vi "ALLPROPS20dll.vi"(8 "error in (no error)":errorcluster, 11 "Inputs":T1) -> (0 "error out":errorcluster, 3 "Outputs":T2)   [LabVIEW 2021]
doc: "subroutine ALLPROPSdll(hOut, iUnits, iMass, iFlag, T, D, zm, Output, hUnits, iUCodeArray, ierr,\nherr, hOut_length, hUnits_length, herr_length)\n\nCalculate the single-phase properties identified in the hOut string at the temperature, density, and composition\nsent to the routine. Return the properties in mass or molar units depending on iUnits.\n\nWarning Do NOT call this routine for two-phase states, otherwise it will return metastable states if near but\ninside the phase boundary, or complete nonsense at other conditions. The value of q that is returned from the\nflash routines will indicate a two phase state by returning a value between 0 and 1. In such a situation, properties\ncan only be calculated for the saturated liquid and vapor states.\n\nFor example, when calling PHFLSH: call subroutine PHFLSH (P,h,z,T,D,Dl,Dv,x,y,q,e,s,Cv,Cp,w,ierr,herr) If q>0 and q<1,\n then values of the liquid and vapor compositions will be returned in the x and y arrays, and the properties of the \nliquid and vapor states can be calculated, for example:\n\ncall ENTRO (T,Dl,x,sliq)\ncall ENTRO (T,Dv,x,svap)\n\nINPUTS:\nhOut -- Input string of properties to calculate (of any length). Inputs can be\nseparated by spaces, commas, semicolons, or bars, but should not be mixed. For example,\na proper string would be hOut=’T,P,D,H,E,S’, whereas an improperly defined string would\nbe hOut=’T,P;D H|E,S’. Use of lower or upper case is not important. Some properties will\nreturn multiple values, for example, hOut=’F,Fc,XMOLE’ will return 12 properties for a\nfour component system, these being F(1), F(2), F(3), F(4), Fc(1), Fc(2), etc. To retrieve the\nproperty of a single component, use, for example, hOut=’XMOLE(2),XMOLE(3)’\niUnits -- See subroutine REFPROP for a complete description of the iUnits input\nvalue. A negative value for iUnits indicates that the input temperature is given in K and\ndensity in mol/dm^3, (Refprop default units), otherwise T and D will be converted first to K\nand mol/dm^3. Do not use the negative value for the iUnits parameter everywhere, only in\nthis one situation.\niMass -- Specifies if the input composition is mole or mass based.\n 0 Input compositions given in mole fractions\n 1 Input compositions given in mass fractions\niFlag -- Turn on or off writing of labels and units to hUnitsArray.\n 0 Do not write anything to the hUnitsArray array, thus increasing the calculation speed. (String handling in \n Fortran is very computationally expensive.)\n 1 Write labels and units to the hUnitsArray array.\n 2 Return only the string number described under “iUCodeArray” below and the units. (No properties will be \n calculated.)\n -1 Write labels and units for only the first item\nT -- Temperature, with units based on the value of iUnits.\nD -- Density, with units based on the value of iUnits.\nz -- Composition on a mole or mass basis (array of size ncmax=20)\n\nOUTPUTS:\nOutput -- Array of properties that were specified in the hOut string. (array\nof size 200 dimensioned as double precision) The number -9999970 will be returned when\nerrors occur or no input was requested.\nhUnits -- String with units. Will also contain error messages when necessary. The string will be empty if iFlag=0.\niUCodeArray -- Array (of size 200) with the values of iUCode(n) described\nin the REFPROP subroutine.\nierr -- Error flag\nherr -- Error string (character*255)\nhOut_length -- length of variable hOut (default: 255)\nhUnits_length -- length of variable hUnits (default: 1000)\nherr_length -- length of variable herr (default: 255)\n\nThe dimension statements for these variables are (in Fortran):\nparameter (ncmax=20) ! Maximum number of components in the mixture\nparameter (iPropMax=200) ! Number of output properties available in ALLPROPS.\ncharacter*10000 hOut ! hOut can actually be of any length.\ncharacter herr*255,hUnitsArray(iPropMax)*50\ninteger ierr,iUnits,iMass,iFlag,iUCodeArray(iPropMax) ! Note: as integer*4\ndouble precision Tx,Dx,zm(ncmax),Output(iPropMax)"
uses:
  REFPROP.dll
panel:
  # "REFPROP-ALLPROPS20dll"
  # "void  ALLPROPS20dll(CStr hOut, int32_t *iUnits, int32_t *iMass, int32_t *iFlag, double *T, double *D, double *z, double *Output, CStr hUnits, int32_t *iUCodeArray, int32_t *ierr, CStr herr, int32_t *hOut_Length, int32_t *hUnitsArray_length, int32_t *herr_length);"
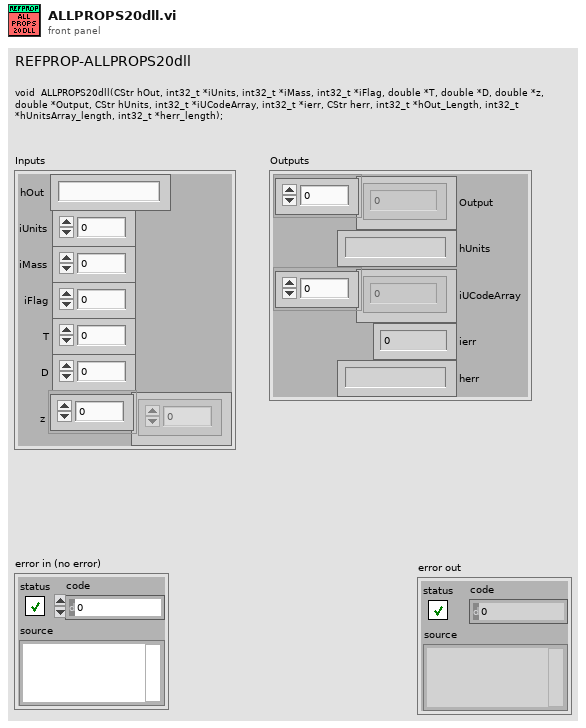
[diagram p1: front panel]
types:
  T1 = cluster{"hOut":string, "iUnits":i32, "iMass":i32, "iFlag":i32, "T":dbl, "D":dbl, "z":dbl[]}
  T2 = cluster{"Output":dbl[], "hUnits":string, "iUCodeArray":i32[], "ierr":i32, "herr":string}
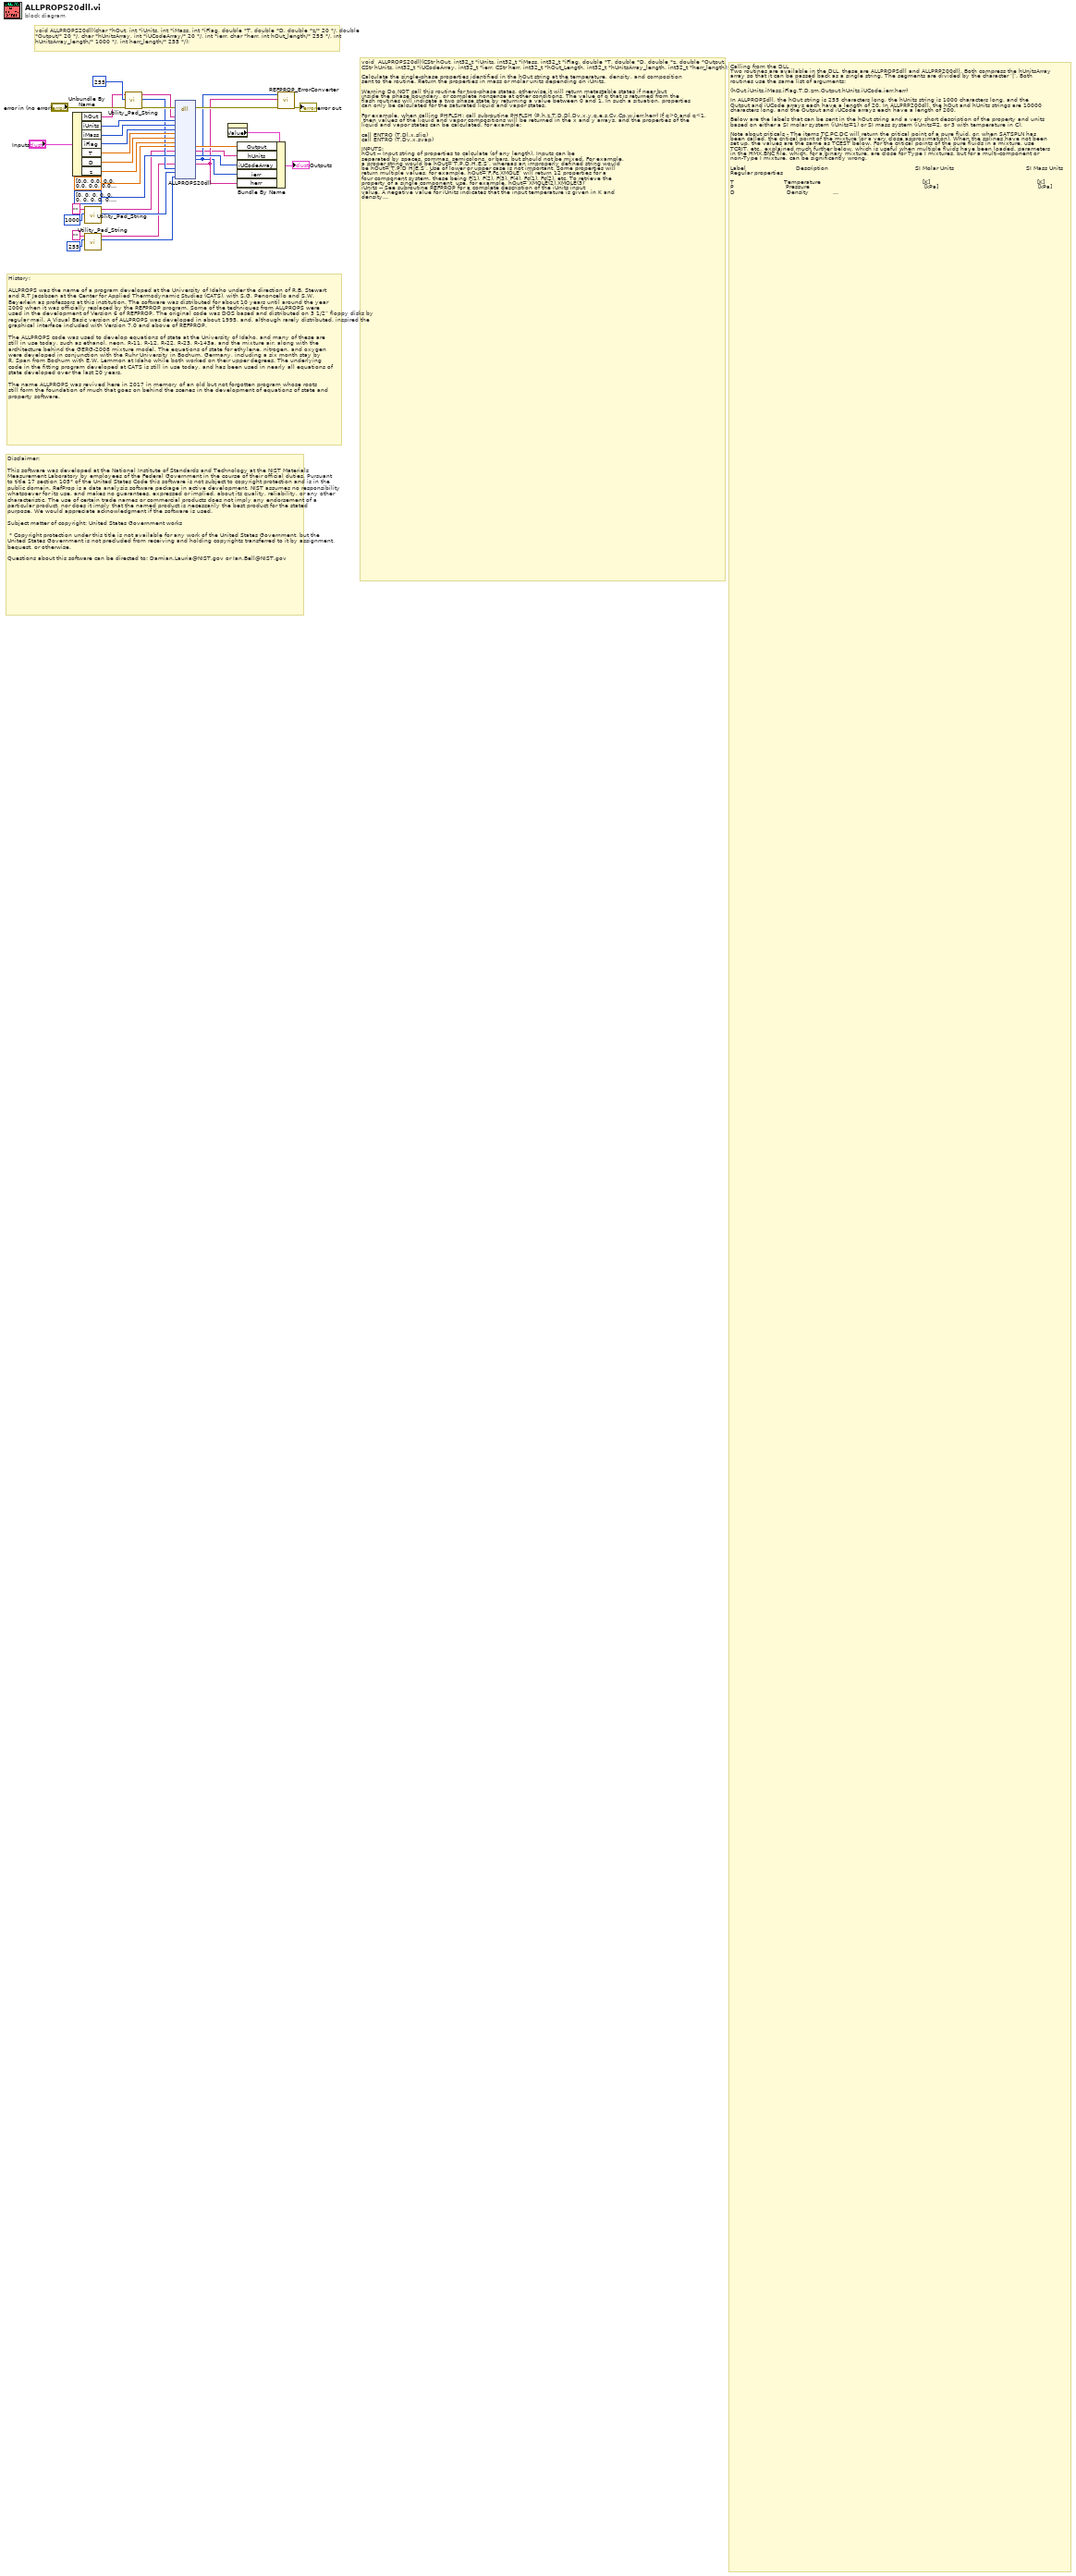
[diagram p0: block diagram]
diagram:
  # "void ALLPROPS20dll(char *hOut, int *iUnits, int *iMass, int *iFlag, double *T, double *D, double *z/* 20 */, double *Output/* 20 */, char *hUnitsArray, int *iUCodeArray/* 20 */, int *ierr, char *herr, int hOut_length/* 255 */, int hUnitsArray_length/* 1000 */, int herr_length/* 255 */);"
  # "Calling from the DLL\nTwo routines are available in the DLL, these are ALLPROPSdll and ALLPRP200dll. Both compress the hUnitsArray\narray so that it can be passed back as a single string. The segments are divided by the character ‘|’. Both\nroutines use the same list of arguments:\n\n(hOut,iUnits,iMass,iFlag,T,D,zm,Output,hUnits,iUCode,ierr,herr)\n\nIn ALLPROPSdll, the hOut string is 255 characters long, the hUnits string is 1000 characters long, and the\nOutput and iUCode arrays each have a length of 20. In ALLPRP200dll, the hOut and hUnits strings are 10000\ncharacters long, and the Output and iUCode arrays each have a length of 200.\n\nBelow are the labels that can be sent in the hOut string and a very short description of the property and units\nbased on either a SI molar system (iUnits=1) or SI mass system (iUnits=2, or 3 with temperature in C).\n\nNote about criticals - The items TC,PC,DC will return the critical point of a pure fluid, or, when SATSPLN has\nbeen called, the critical point of the mixture (or a very close approximation). When the splines have not been\nset up, the values are the same as TCEST below. For the critical points of the pure fluids in a mixture, use\nTCRIT, etc., explained much further below, which is useful when multiple fluids have been loaded. parameters\nin the HMX.BNC file, which, for a binary mixture, are close for Type I mixtures, but for a multi-component or\nnon-Type I mixture, can be significantly wrong.\n\nLabel                           Description                                               SI Molar Units                                       SI Mass Units\nRegular properties\n\nT                           Temperature                                                       [K]                                                          [K]\nP                            Pressure                                                              [kPa]                                                      [kPa]\nD                            Density                                                               [mol/dm^3]                                         [kg/m^3]\nV                            Volume                                                               [dm^3/mol]                                         [m^3/kg]\nE                            Internal energy                                                   [J/mol]                                                  [kJ/kg]\nH                           Enthalpy                                                              [J/mol]                                                  [kJ/kg]\nS                            Entropy                                                                [J/(mol*K)]                                           [(kJ/kg)/K]\nCV                          Isochoric heat capacity                                    [J/(mol*K)]                                           [(kJ/kg)/K]\nCP                          Isobaric heat capacity                                      [J/(mol*K)]                                           [(kJ/kg)/K]\nCP/CV                  Heat capacity ratio                                            [-]                                                           [-]\nW                           Speed of sound                                                 [m/s]                                                     [m/s]\nZ                           Compressibility factor                                       [-]                                                           [-]\nJT                          Isenthalpic Joule-Thomson coefficient          [K/kPa]                                                  [K/kPa]\nA                           Helmholtz energy                                              [J/mol]                                                  [kJ/kg]\nG                           Gibbs energy                                                       [J/mol]                                                  [kJ/kg]\nR                           Gas constant                                                        [J/(mol*K)]                                           [(kJ/kg)/K]\nM                           Molar mass (or of the mixture)                        [g/mol]                                                 [g/mol]\nQ                           Quality (not implemented, q not known)       [mol/mol]                                            [kg/kg]\n\nNot so regular properties\n\nKAPPA                  Isothermal compressibility                                [1/kPa]                                                  [1/kPa]\nBETA                     Volume expansivity                                            [1/K]                                                      [1/K]\nISENK                    Isentropic expansion coefficient                       [-]                                                          [-]\nKT                          Isothermal expansion coefficient                     [-]                                                          [-]\nBETAS                   Adiabatic compressibility                                  [1/kPa]                                                  [1/kPa]\nBS                          Adiabatic bulk modulus                                    [kPa]                                                      [kPa]\nKKT                        Isothermal bulk modulus                                  [kPa]                                                     [kPa]\nTHROTT                Isothermal throttling coefficient                     [dm^3/mol]                                         [m^3/kg]\n\nDerivatives\n\nDPDD                      dP/dD at constant T                                         [(dm^3/mol)*kPa]                               [(m^3/kg)*kPa]\nDPDT                      dP/dT at constant D                                         [kPa/K]                                                   [kPa/K]\nDDDP                      dD/dP at constant T                                         [(mol/dm^3)/kPa]                               [(kg/m^3)/kPa]\nDDDT                      dD/dT at constant P                                         [(mol/dm^3)/K]                                   [(kg/m^3)/K]\nDTDP                      dT/dP at constant D                                         [K/kPa]                                                   [K/kPa]\nDTDD                      dT/dD at constant P                                         [(dm^3/mol)*K]                                   [(m^3/kg)*K]\nD2PDD2                  d^2P/dD^2 at constant T                                [(dm^3/mol)^2*kPa]                          [(m^3/kg)^2*kPa]\nD2PDT2                  d^2P/dT^2 at constant D                                [kPa/K^2]                                              [kPa/K^2]\nD2PDTD                 d^2P/dTdD                                                         [(dm^3/mol)*kPa/K]                          [(m^3/kg)*kPa/K]\nD2DDP2                 d^2D/dP^2 at constant T                                 [(mol/dm^3)/kPa^2]                          [(kg/m^3)/kPa^2]\nD2DDT2                  d^2D/dT^2 at constant P                                [(mol/dm^3)/K^2]                              [(kg/m^3)/K^2]\nD2DDPT                  d^2D/dPdT                                                        [(mol/dm^3)/(kPa*K)]                        [(kg/m^3)/[kPa*K]]\nD2TDP2                  d^2T/dP^2 at constant D                                 [K/kPa^2]                                             [K/kPa^2]\nD2TDD2                  d^2T/dD^2 at constant P                                 [(dm^3/mol)^2*K]                             [(m^3/kg)^2*K]\nD2TDPD                  d^2T/dPdD                                                        [(dm^3/mol)*K/kPa]                           [(m^3/kg)*K/kPa]\n\nEnthalpy derivatives\n\nDHDT_D                 dH/dT at constant D                                          [(J/mol)/K]                                            [(kJ/kg)/K]\nDHDT_P                 dH/dT at constant P                                           [(J/mol)/K]                                            [(kJ/kg)/K]\nDHDD_T                 dH/dD at constant P                                          [(J/mol)*(dm^3/mol)]                        [(kJ/kg)*(m^3/kg)]\nDHDD_P                 dH/dD at constant T                                          [(J/mol)*(dm^3/mol)]                        [(kJ/kg)*(m^3/kg)]\nDHDP_T                 dH/dP at constant T                                           [(J/mol)/kPa]                                        [(kJ/kg)/kPa]\nDHDP_D                 dH/dP at constant D                                          [(J/mol)/kPa]                                        [(kJ/kg)/kPa]\n\nEntropy derivatives\n\nDSDT_D                  dS/dT at constant D                                             [(J/mol)/K^2]                                      [(kJ/kg)/K^2]\nDSDT_P                  dS/dT at constant P                                             [(J/mol)/K^2]                                       [(kJ/kg)/K^2]\nDSDD_T                  dS/dD at constant T                                             [(J/mol)*(dm^3/mol)/K]                   [(kJ/kg)*(m^3/kg)/K]\nDSDD_P                  dS/dD at constant P                                             [(J/mol)*(dm^3/mol)/K]                   [(kJ/kg)*(m^3/kg)/K]\nDSDP_T                  dS/dP at constant T                                             [(J/mol)/(kPa*K)]                                 [(kJ/kg)/[kPa*K]]\nDSDP_D                  dS/dP at constant D                                             [(J/mol)/(kPa*K)]                                [(kJ/kg)/[kPa*K]]\n\nVirial Coefficients\n\nXB                           Second virial coefficient                                      [dm^3/mol]                                        [m^3/kg]\nXC                           Third virial coefficient                                          [(dm^3/mol)^2]                                [(m^3/kg)^2]\nXD                           Fourth virial coefficient                                       [(dm^3/mol)^3]                                 [(m^3/kg)^3]\nXE                            Fifth virial coefficient                                           [(dm^3/mol)^4]                                [(m^3/kg)^4]\nXBXT                       1st derivative of B with respect to T                   [(dm^3/mol)/K]                                [(m^3/kg)/K]\nX2BXT2                   2nd derivative of B with respect to T                 [(dm^3/mol)/K^2]                            [(m^3/kg)/K^2]\nXCXT                       1st derivative of C with respect to T                  [(dm^3/mol)^2/K]                            [(m^3/kg)^2/K]\nX2CXT2                   2nd derivative of C with respect to T                [(dm^3/mol)^2/K^2]                        [(m^3/kg)^2/K^2]\nXDXT                       1st derivative of D with respect to T                  [(dm^3/mol)^3/K]                            [(m^3/kg)^3/K]\nX2DXT2                   2nd derivative of D with respect to T                [(dm^3/mol)^3/K^2]                        [(m^3/kg)^3/K^2]\nBA                            Second acoustic virial coefficient                      [dm^3/mol]                                       [m^3/kg]\nCA                            Third acoustic virial coefficient                         [(dm^3/mol)^2]                                [(m^3/kg)^2]\n\nEOS testing properties\n\nGRUN                       Gruneisen parameter                                          [-]                                                        [-]\nPIP                            Phase identification parameter                         [-]                                                        [-]\nRIEM                        Thermodyn. curvature (nm^3/mol)\n(Z-1)/D                     (Z-1) over the density                                         [dm^3/mol]                                     [m^3/kg]\n(Z-1)/P                     (Z-1) over the pressure                                       [1/kPa]                                               [1/kPa]\nP*V                           Pressure times volume                                       [(dm^3/mol)*kPa]                           [(m^3/kg)*kPa]\nS*D                           Entropy times density                                         [J/(mol*K)*(mol/dm^3)]                [(kJ/kg)*(kg/m^3)/K]\nN1/T                        Negative reciprocal temperature                       [1/K]                                                  [1/K]\nRD                            Rectilinear diameter (Dl+Dv)/2                          [mol/dm^3]                                     [kg/m^3]\n\nProperties from ancillary equations\n\nANC-TP                   Vapor pressure from ancillary given T             [kPa]                                                  [kPa]\nANC-TDL                 Sat. liquid dens. from ancillary given T           [mol/dm^3]                                     [kg/m^3]\nANC-TDV                 Sat. vapor dens. from ancillary given T           [mol/dm^3]                                     [kg/m^3]\nANC-PT                    Vapor temp. from ancillary given P                 [K]                                                     [K]\nANC-DT                    Vapor temp. from ancillary given D                [K]                                                     [K]\nMELT-TP                  Melting pressure given T                                   [kPa]                                                 [kPa]\nMELT-PT                  Melting temperature given P                            [K]                                                     [K]\nSUBL-TP                   Sublimation pressure given T                           [kPa]                                                 [kPa]\nSUBL-PT                   Sublimation temperature given P                    [K]                                                     [K]\n\nLess common saturation properties\n\nCSAT                        Saturated heat capacity                                       [J/(mol*K)]                                     [(kJ/kg)/K]\nCV2P                         Isochoric two-phase heat capacity                   [J/(mol*K)]                                     [(kJ/kg)/K]\nDPDTSAT                 dP/dT along the saturation line                         [kPa/K]                                           [kPa/K]\nDHDZSAT                dH/dZ along the sat. line (Waring)                    [J/mol]                                            [kJ/kg]\nLIQSPNDL                Density at the liquid spinodal                             [mol/dm^3]                                  [kg/m^3]\nVAPSPNDL               Density at the vapor spinodal                            [mol/dm^3]                                   [kg/m^3]\n\nExcess properties\n\nVE                             Excess volume                                                       [dm^3/mol]                                  [m^3/kg]\nEE                             Excess energy                                                         [J/mol]                                           [kJ/kg]\nHE                            Excess enthalpy                                                      [J/mol]                                           [kJ/kg]\nSE                             Excess entropy                                                       [J/(mol*K)]                                     [(kJ/kg)/K]\nAE                            Excess Helmholtz energy                                      [J/mol]                                           [kJ/kg]\nGE                            Excess Gibbs energy                                              [J/mol]                                           [kJ/kg]\nB12                          B12                                                                           [dm^3/mol]                                  [m^3/kg]\n\nIdeal gas properties\n\nP0                            Ideal gas pressure                                                   [kPa]                                                [kPa]\nE0                            Ideal gas internal energy                                        [J/mol]                                            [kJ/kg]\nH0                           Ideal gas enthalpy                                                   [J/mol]                                            [kJ/kg]\nS0                            Ideal gas entropy                                                    [J/(mol*K)]                                      [(kJ/kg)/K]\nCV0                         Ideal gas isochoric heat capacity                          [J/(mol*K)]                                     [(kJ/kg)/K]\nCP0                         Ideal gas isobaric heat capacity                            [J/(mol*K)]                                     [(kJ/kg)/K]\nCP0/CV0                Ideal gas heat capacity ratio                                  [-]                                                    [-]\nW0                          Ideal gas speed of sound                                        [m/s]                                              [m/s]\nA0                           Ideal gas Helmholtz energy                                    [J/mol]                                           [kJ/kg]\nG0                           Ideal gas Gibbs energy                                            [J/mol]                                           [kJ/kg]\nP-P0                       Pressure minus ideal gas pressure                         [kPa]                                               [kPa]\n\nResidual properties\n\nPR                         Residual pressure (P-D*Rxgas*T)                             [kPa]                                              [kPa]\nER                         Residual internal energy                                            [J/mol]                                          [kJ/kg]\nHR                        Residual enthalpy                                                       [J/mol]                                          [kJ/kg]\nSR                         Residual entropy                                                        [J/(mol*K)]                                    [(kJ/kg)/K]\nCVR                      Residual isochoric heat capacity                              [J/(mol*K)]                                   [(kJ/kg)/K]\nCPR                      Residual isobaric heat capacity                                [J/(mol*K)]                                    [(kJ/kg)/K]\nAR                        Residual Helmholtz energy                                       [J/mol]                                           [kJ/kg]\nGR                        Residual Gibbs energy                                                [J/mol]                                          [kJ/kg]\n\nIdeal-gas contributions to the Helmholtz energy\n\nPHIG00                    Red. IG Helmholtz energy A0/RT                         [-]                     \t                            [-]\nPHIG10                    tau*[d(A0/RT)/d(tau)]                                           [-]                     \t                            [-]\nPHIG20                    tau^2*[d^2(A0/RT)/d(tau)^2]                             [-]                     \t                            [-]\nPHIG30                    tau^3*[d^3(A0/RT)/d(tau)^3]                             [-]                     \t                            [-]\nPHIG01                    del*[d(A0/RT)/d(del)]                                            [-]                     \t                            [-]\nPHIG02                    del^2*[d^2(A0/RT)/d(del)^2]                              [-]                     \t                            [-]\nPHIG03                    del^3*[d^3(A0/RT)/d(del)^3]                              [-]                     \t                            [-]\nPHIG11                    tau*del*[d^2(A0/RT)/d(tau)d(del)]                     [-]                     \t                            [-]\nPHIG12                    tau*del^2*[d^3(A0/RT)/d(tau)d(del)^2]            [-]                     \t                            [-]\nPHIG21                    tau^2*del*[d^3(A0/RT)/d(tau)^2d(del)]            [-]                     \t                            [-]\n\nResidual contributions to the Helmholtz energy\n\nPHIR00                    Red. resid. Helmholtz energy Ar/RT                    [-]                                                  [-]\nPHIR10                    tau*[d(Ar/RT)/d(tau)]                                \t\t\t         [-]                                                  [-]\nPHIR20                    tau^2*[d^2(Ar/RT)/d(tau)^2]                          \t\t\t [-]                                                  [-]\nPHIR30                    tau^3*[d^3(Ar/RT)/d(tau)^3]                          \t\t\t [-]                                                  [-]\nPHIR01                    del*[d(Ar/RT)/d(del)]                                \t\t\t          [-]                                                  [-]\nPHIR02                    del^2*[d^2(Ar/RT)/d(del)^2]                          \t\t\t  [-]                                                  [-]\nPHIR03                    del^3*[d^3(Ar/RT)/d(del)^3]                          \t\t\t  [-]                                                  [-]\nPHIR11                    tau*del*[d^2(Ar/RT)/d(tau)d(del)]                    \t\t[-]                                                  [-]\nPHIR12                    tau*del^2*[d^3(Ar/RT)/d(tau)d(del)^2]             [-]                                                  [-]\nPHIR21                    tau^2*del*[d^3(Ar/RT)/d(tau)^2d(del)]             [-]                                                  [-]\n\nCritical point and P,T maximums along isopleth (see above)\n\nTC                           Critical temperature of a pure fluid                      [K]                                                  [K]\nPC                           Critical pressure of a pure fluid                             [kPa]                                              [kPa]\nDC                           Critical density of a pure fluid                               [mol/dm^3]                                 [kg/m^3]\nTCEST                     Estimated critical temperature                              [K]                                                  [K]\nPCEST                     Estimated critical temperature                              [kPa]                                              [kPa]\nDCEST                     Estimated critical density                                       [mol/dm^3]                                 [kg/m^3]\nTMAXT                   Temperature at cricondentherm                           [K]                                                  [K]\nPMAXT                   Pressure at cricondentherm                                   [kPa]                                              [kPa]\nDMAXT                   Density at cricondentherm                                    [mol/dm^3]                                 [kg/m^3]\nTMAXP                   Temperature at cricondenbar                                [K]                                                  [K]\nPMAXP                   Pressure at cricondenbar                                        [kPa]                                              [kPa]\nDMAXP                   Density at cricondenbar                                         [mol/dm^3]                                 [kg/m^3]\n\nReducing parameters\n\nTRED                       Reducing temperature                                           [K]                                                 [K]\nDRED                       Reducing density                                                    [mol/dm^3]                                [kg/m^3]\nTAU                         Tc/T (or Tred/T)                                                      [-]                                                 [-]\nDEL                          D/Dc (or D/Dred)                                                     [-]                                                 [-]\n\nLimits\n\nTMIN                       Minimum temperature of the EOS                       [K]                                                [K]\nTMAX                      Maximum temperature of the EOS                       [K]                                                [K]\nDMAX                      Maximum density of the EOS                                [mol/dm^3]                              [kg/m^3]\nPMAX                      Maximum pressure of the EOS                              [kPa]                                            [kPa]\n\nTransport, etc.\n\nVIS                           Viscosity                                                                    [uPa*s]                                        [uPa*s]\nTCX                         Thermal conductivity                                              [W/(m*K)]                                  [W/(m*K)]\nPRANDTL               Prandlt number                                                        [-]                                                [-]\nTD                           Thermal diffusivity                                                   [cm^2/s]                                    [cm^2/s]\nKV                           Kinematic Viscosity                                                  [cm^2/s]                                    [cm^2/s]\nSTN                        Surface tension                                                          [mN/m]                                     [mN/m]\nDE                           Dielectric constant                                                    [-]                                                [-]\n\nHeating values\n\nSPHT                      Specific heat input                                                    [J/mol]                                       [kJ/kg]\nHFRM                     Heat of formation                                                     [J/mol]                                       [kJ/kg]\nHG                          Gross (or superior) heating value                            [J/mol]                                       [kJ/kg]\nHN                          Net (or inferior) heating value                                 [J/mol]                                       [kJ/kg]\nHGLQ                     Gross Heat. Val. (Liquid)                                           [J/mol]                                       [kJ/kg]\nHNLQ                     Net Heat. Val. (Liquid)                                              [J/mol]                                       [kJ/kg]\nHGVOL                   Gross HV (Ideal gas volume basis)                          [MJ/m^3]                                  [MJ/m^3]\nHNVOL                   Net HV (Ideal gas volume basis)                             [MJ/m^3]                                  [MJ/m^3]\nHEATVAP               Heat of vaporization (for pure fluids)                     [J/mol]                                       [kJ/kg]\nHEATVAP_T           ...at constant temperature (for mixtures)               [J/mol]                                       [kJ/kg]\nHEATVAP_P           ...at constant pressure (for mixtures)                      [J/mol]                                       [kJ/kg]\nHEATVALUE           Heating value (mass or molar basis)\n\nOther properties\n\nPINT                        Internal pressure                                                       [kPa]                                            [kPa]\nPREP                        Repulsive part of pressure                                       [kPa]                                            [kPa]\nPATT                       Attractive part of pressure                                       [kPa]                                            [kPa]\nEXERGY                   Flow Exergy                                                                [J/mol]                                        [kJ/kg]\nCEXERGY                Closed System Exergy                                               [J/mol]                                        [kJ/kg]\nCSTAR                    Critical flow factor                                                     [-]                                                 [-]\nTMF                        Throat mass flux                                                        [kg/(m^2*s)]                              [kg/(m^2*s)]\nFPV                          Supercompressibility                                                [-]                                                 [-]\nSUMFACT               Summation Factor                                                    [-]                                                 [-]\nRDAIR                      Relative Density in air (specific gravity)                 [-]                                                 [-]\nRDH2O                    Relative Density in water (specific gravity)            [-]                                                 [-]\nAPI                           API Gravity                                                                 [-]                                                 [-]\n\nFluid fixed points for mixtures \nAt the “true” critical point of the EOS dP/dD=0 and d^P/dD^2=0 at constant temperature\n\nTCRIT                     Critical temperature of component i                       [K]                                                [K]\nPCRIT                     Critical pressure of component i                              [kPa]                                            [kPa]\nDCRIT                     Critical density of component i                                [mol/dm^3]                               [kg/m^3]\nTTRP                      Triple point temperature of component i                [K]                                                [K]\nPTRP                      Triple point pressure of component i                       [kPa]                                            [kPa]\nDTRP                      Triple point density of component i                         [mol/dm^3]                               [kg/m^3]\nTNBP                      Normal boiling point temp. of comp. i                    [K]                                                [K]\nREOS                      Gas constant of component i for EOS                       [J/(mol*K)]                                  [(kJ/kg)/K]\nMM                        Molar mass of component i                                       [g/mol]                                        [g/mol]\nACF                        Acentric factor of component i                                 [-]                                                  [-]\nDIPOLE                  Dipole moment of component i                                [debye]                                        [debye]\nTREF                      Ref. state temperature of component i                     [K]                                                 [K]\nDREF                      Ref. state pressure of component i                            [kPa]                                             [kPa]\nHREF                      Ref. state enthalpy of comp. i at T0 and P0              [J/mol]                                         [kJ/kg]\nSREF                       Ref. state entropy of comp. i at T0 and P0                [J/(mol*K)]                                  [(kJ/kg)/K]\n\nTransport properties as a function of component number\nViscosity=ETA0+ETAB2+ETAR+ETAC\nThermal conductivity=TCX0+TCXR+TCXC\n\nETA0                     Dilute gas viscosity of component i                            [uPa*s]                                         [uPa*s]\nETAB2                   2nd virial viscosity of component i                             [uPa*s]                                         [uPa*s]\nETAR                     Residual viscosity of component i                               [uPa*s]                                        [uPa*s]\nETAC                    Viscosity critical enhance. of comp. i                          [uPa*s]                                         [uPa*s]\nTCX0                     Dilute gas thermal cond. of comp. i                            [W/(m*K)]                                   [W/(m*K)]\nTCXR                     Residual (background) cond. of comp. i                    [W/(m*K)]                                   [W/(m*K)]\nTCXC                    Cond. crit. enhancement of comp. i                            [W/(m*K)]                                   [W/(m*K)]\n\nMixture properties as a function of component number\n\nK                            K value (y/x) (not implemented, y unknown)             [-]                                                 [-]\nF                            Fugacities                                                                         [kPa]                                             [kPa]\nFC                         Fugacity coefficients                                                       [-]                                                 [-]\nCPOT                   Chemical potentials                                                         [J/mol]                                        [kJ/kg]\nDADN                  n*partial(alphar)/partial(ni)                                             [-]                                                [-]\nDNADN               partial(n*alphar)/partial(ni)                                             [-]                                                [-]\nXMOLE                Composition on a mole basis                                         [-]                                                [-]\nXMASS                Composition on a mass basis                                         [-]                                                [-]\nFIJMIX                  Binary parameters (see REFPROP)"
  # "void  ALLPROPS20dll(CStr hOut, int32_t *iUnits, int32_t *iMass, int32_t *iFlag, double *T, double *D, double *z, double *Output, \nCStr hUnits, int32_t *iUCodeArray, int32_t *ierr, CStr herr, int32_t *hOut_Length, int32_t *hUnitsArray_length, int32_t *herr_length);\n\nCalculate the single-phase properties identified in the hOut string at the temperature, density, and composition\nsent to the routine. Return the properties in mass or molar units depending on iUnits.\n\nWarning Do NOT call this routine for two-phase states, otherwise it will return metastable states if near but\ninside the phase boundary, or complete nonsense at other conditions. The value of q that is returned from the\nflash routines will indicate a two phase state by returning a value between 0 and 1. In such a situation, properties\ncan only be calculated for the saturated liquid and vapor states.\n\nFor example, when calling PHFLSH: call subroutine PHFLSH (P,h,z,T,D,Dl,Dv,x,y,q,e,s,Cv,Cp,w,ierr,herr) If q>0 and q<1,\n then values of the liquid and vapor compositions will be returned in the x and y arrays, and the properties of the \nliquid and vapor states can be calculated, for example:\n\ncall ENTRO (T,Dl,x,sliq)\ncall ENTRO (T,Dv,x,svap)\n\nINPUTS:\nhOut -- Input string of properties to calculate (of any length). Inputs can be\nseparated by spaces, commas, semicolons, or bars, but should not be mixed. For example,\na proper string would be hOut=’T,P,D,H,E,S’, whereas an improperly defined string would\nbe hOut=’T,P;D H|E,S’. Use of lower or upper case is not important. Some properties will\nreturn multiple values, for example, hOut=’F,Fc,XMOLE’ will return 12 properties for a\nfour component system, these being F(1), F(2), F(3), F(4), Fc(1), Fc(2), etc. To retrieve the\nproperty of a single component, use, for example, hOut=’XMOLE(2),XMOLE(3)’\niUnits -- See subroutine REFPROP for a complete description of the iUnits input\nvalue. A negative value for iUnits indicates that the input temperature is given in K and\ndensity in mol/dm^3, (Refprop default units), otherwise T and D will be converted first to K\nand mol/dm^3. Do not use the negative value for the iUnits parameter everywhere, only in\nthis one situation.\niMass -- Specifies if the input composition is mole or mass based.\n                0 Input compositions given in mole fractions\n                1 Input compositions given in mass fractions\niFlag -- Turn on or off writing of labels and units to hUnitsArray.\n              0 Do not write anything to the hUnitsArray array, thus increasing the calculation speed. (String handling in  \n              Fortran is very computationally expensive.)\n              1 Write labels and units to the hUnitsArray array.\n              2 Return only the string number described under “iUCodeArray” below and the units. (No properties will be \n              calculated.)\n            -1 Write labels and units for only the first item\nT -- Temperature, with units based on the value of iUnits.\nD -- Density, with units based on the value of iUnits.\nz -- Composition on a mole or mass basis (array of size ncmax=20)\n\nOUTPUTS:\nOutput -- Array of properties that were specified in the hOut string. (array\nof size 200 dimensioned as double precision) The number -9999970 will be returned when\nerrors occur or no input was requested.\nhUnits -- String with units. Will also contain error messages when necessary. The string will be empty if iFlag=0.\niUCodeArray -- Array (of size 200) with the values of iUCode(n) described\nin the REFPROP subroutine.\nierr -- Error flag\nherr -- Error string (character*255)\nhOut_length -- length of variable hOut (default: 255)\nhUnits_length -- length of variable hUnits (default: 1000)\nherr_length -- length of variable herr (default: 255)\n\nThe dimension statements for these variables are (in Fortran):\nparameter (ncmax=20) ! Maximum number of components in the mixture\nparameter (iPropMax=200) ! Number of output properties available in ALLPROPS.\ncharacter*10000 hOut ! hOut can actually be of any length.\ncharacter herr*255,hUnitsArray(iPropMax)*50\ninteger ierr,iUnits,iMass,iFlag,iUCodeArray(iPropMax) ! Note: as integer*4\ndouble precision Tx,Dx,zm(ncmax),Output(iPropMax)"
  # "History:\n\nALLPROPS was the name of a program developed at the University of Idaho under the direction of R.B. Stewart\nand R.T Jacobsen at the Center for Applied Thermodynamic Studies (CATS), with S.G. Penoncello and S.W.\nBeyerlein as professors at this institution. The software was distributed for about 10 years until around the year\n2000 when it was officially replaced by the REFPROP program. Some of the techniques from ALLPROPS were\nused in the development of Version 6 of REFPROP. The original code was DOS based and distributed on 3 1/2” floppy disks by regular mail. A Visual Basic version of ALLPROPS was developed in about 1995, and, although rarely distributed, inspired the graphical interface included with Version 7.0 and above of REFPROP.\n\nThe ALLPROPS code was used to develop equations of state at the University of Idaho, and many of these are\nstill in use today, such as ethanol, neon, R-11, R-12, R-22, R-23, R-143a, and the mixture air, along with the\narchitecture behind the GERG-2008 mixture model. The equations of state for ethylene, nitrogen, and oxygen\nwere developed in conjunction with the Ruhr University in Bochum, Germany, including a six month stay by\nR. Span from Bochum with E.W. Lemmon at Idaho while both worked on their upper degrees. The underlying\ncode in the fitting program developed at CATS is still in use today, and has been used in nearly all equations of\nstate developed over the last 20 years.\n\nThe name ALLPROPS was revived here in 2017 in memory of an old but not forgotten program whose roots\nstill form the foundation of much that goes on behind the scenes in the development of equations of state and\nproperty software."
  # "Disclaimer:\n\nThis software was developed at the National Institute of Standards and Technology at the NIST Materials Measurement Laboratory by employees of the Federal Government in the course of their official duties. Pursuant to title 17 section 105* of the United States Code this software is not subject to copyright protection and is in the public domain. RefProp is a data analysis software package in active development. NIST assumes no responsibility whatsoever for its use, and makes no guarantees, expressed or implied, about its quality, reliability, or any other characteristic. The use of certain trade names or commercial products does not imply any endorsement of a particular product, nor does it imply that the named product is necessarily the best product for the stated purpose. We would appreciate acknowledgment if the software is used.\n \nSubject matter of copyright: United States Government works\n  \n * Copyright protection under this title is not available for any work of the United States Government, but the United States Government is not precluded from receiving and holding copyrights transferred to it by assignment, bequest, or otherwise.\n\nQuestions about this software can be directed to: Damian.Lauria@NIST.gov or Ian.Bell@NIST.gov"
  n1 = Unbundle By Name("Inputs") -> ("hOut"=w11:string, "iUnits"=w27:i32, "iMass"=w26:i32, "iFlag"=w25:i32, "T"=w24:dbl, "D"=w23:dbl, "z"=w22:dbl[])
  n2 = call "Utility_Pad_String.vi"("Target Length"=1000, "String in"="") -> ("Length out"=w3:i32, "result string"=w4:string)  [unwired: 7 in, 1 out]
  n3 = call "Utility_Pad_String.vi"("Target Length"=255, "String in"="") -> ("Length out"=w1:i32, "result string"=w2:string)  [unwired: 7 in, 1 out]
  n4 = call "Utility_Pad_String.vi"("error in (no error)"="error in (no error)", "Target Length"=255, "String in"=w11) -> ("error out"=w12:errorcluster, "Length out"=w9:i32, "result string"=w10:string)  [unwired: 6 in]
  n5 = dll-call lib="C:/Users/lauria/OneDrive - NIST/LabVIEW Projects/7 REFPROP/REFPROP-wrappers-master/REFPROP-wrappers-master/wrappers/LabVIEW/REFPROP/REFPROP.*" fn="ALLPROPS20dll"(error in=w12, "hOut"=w10, "iUnits"=w27, "iMass"=w26, "iFlag"=w25, "T"=w24, "D"=w23, "z"=w22, "Output"=dbl[] [0.0, 0.0, 0.0, 0.0, 0.0, 0.0, 0.0, 0.0, 0.0, 0.0, 0.0, 0.0, 0.0, 0.0, 0.0, 0.0, 0.0, 0.0, 0.0, 0.0], "hUnits"=w4, "iUCodeArray"=i32[] [0, 0, 0, 0, 0, 0, 0, 0, 0, 0, 0, 0, 0, 0, 0, 0, 0, 0, 0, 0], "herr"=w2, "hOut_Length"=w9, "hUnitsArray_length"=w3, "herr_length"=w1) -> (error out=w32:errorcluster, "Output"=w21:dbl[], "hUnits"=w15:string, "iUCodeArray"=w20:i32[], "ierr"=w18:i32, "herr"=w19:string)  [unwired: 14 in, 1 out]
  n6 = property on="Outputs" class="Clust (strict)"() -> ("Value"=w30:T2)  [unwired: 2 in, 2 out]
  n7 = Bundle By Name(cluster=w30, "Output"=w21, "hUnits"=w15, "iUCodeArray"=w20, "ierr"=w18, "herr"=w19) -> (→"Outputs":T2)
  n8 = call "REFPROP_ErrorConverter.vi"("error in (no error)"=w32, "Error Message"=w19, "Error Code"=w18) -> ("error out"=→"error out":errorcluster)  [unwired: 8 in]
